vi "Write AiSampleClkTask.vi"(8 "error in (no error)":errorcluster, 10 "AiSampleClkTask":refnum<k21>, 11 "DaqMx_Single in":refnum<class "DaqMx_Single.lvclass">) -> (0 "error out":errorcluster, 3 "DaqMx_Single out":refnum<class "DaqMx_Single.lvclass">)   [LabVIEW 2014, in "FgenPlugins.lvlib" / "DaqMx_Single.lvclass"]
uses:
  DaqMx_Single.lvclass
  DaqMx_Single.lvclass/DaqMx_Single.ctl
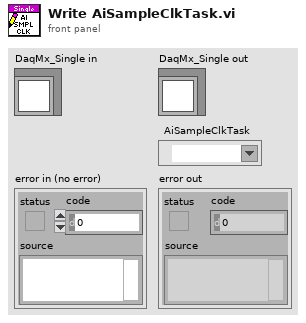
[diagram p1: front panel]
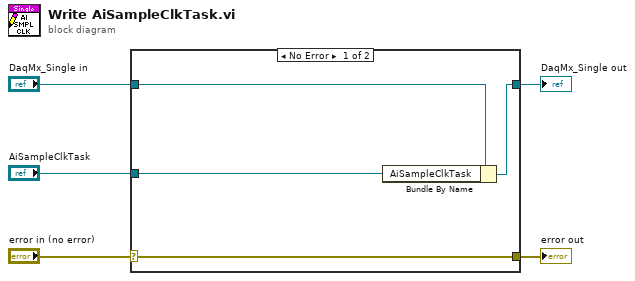
[diagram p0: block diagram]
diagram:
  n1 = case shown="No Error" "error in (no error)" {
    selector: "error in (no error)" -> [w9 w10]
    tunnel: [w9 w10] -> w4
    tunnel: [w7 w11] -> w2
    tunnel: "DaqMx_Single in" -> [w8 w11]
    tunnel: "AiSampleClkTask" -> [w6 _]
    frame No Error {
      n2 = Bundle By Name(cluster=w8, "AiSampleClkTask"=w6) -> (w7:refnum<class "DaqMx_Single.lvclass">)
    }
    frame Error {
    }
  }
  "error out" <- w4
  "DaqMx_Single out" <- w2
